vi "Agilent PSG MXG_Configure RF.vi"(8 "error in":errorcluster, 9 "Level":dbl=-90.0 format="%.2f", 10 "Frequency (Hz)":dbl=100000000.0 format="%.2p", 11 "Handle In":variant) -> (0 "error out":errorcluster {"code" format="%.0x"}, 3 "Handle Out":variant)   [LabVIEW 2015]
uses:
  <instrlib>/Agilent PSG MXG Series/Agilent PSG MXG Series.lvlib
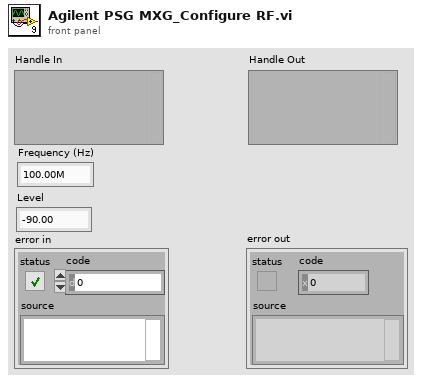
[diagram p1: front panel]
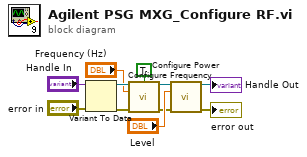
[diagram p0: block diagram]
diagram:
  n1 = Variant To Data(error in="error in", Variant="Handle In") -> (data=w9:refnum<visa-resource-name>, error out=w7:errorcluster)  [unwired: 1 in]
  n2 = call <instrlib>:"Configure Frequency.vi"("VISA resource name"=w9, "Enable Reference Frequency (F:Disable)"=TRUE, "Frequency (100 kHz)"="Frequency (Hz)", "error in (no error)"=w7) -> ("VISA resource name out"=w5:refnum<visa-resource-name>, "error out"=w3:errorcluster)  [unwired: 10 in]
  n3 = call <instrlib>:"Configure Power.vi"("VISA resource name"=w5, "Power (-130 dBm)"="Level", "error in (no error)"=w3) -> ("VISA resource name out"=→"Handle Out":refnum<visa-resource-name>, "error out"=→"error out":errorcluster)  [unwired: 11 in]
